vi "LJM_NameToAddress.vi"(8 "error in":errorcluster, 11 "Name":string) -> (0 "error out":errorcluster, 2 "Type":i32, 3 "Address":i32)   [LabVIEW 2025]
uses:
  labjackm.dll
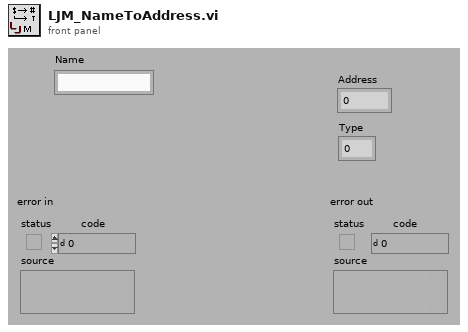
[diagram p1: front panel]
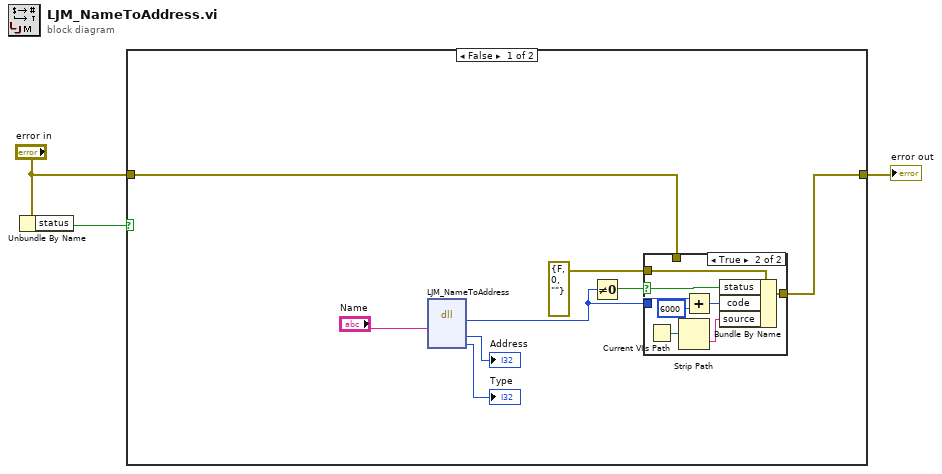
[diagram p0: block diagram]
diagram:
  n1 = Unbundle By Name("error in") -> ("status"=w3:bool)
  n2 = case shown="False" w3 {
    tunnel: "error in" -> [w8 w21]
    tunnel: [w7 w21] -> w1
    frame False {
      n3 = dll-call lib="labjackm.dll" fn="LJM_NameToAddress"("Name"="Name") -> (w11:i32, "Address"=→"Address":i32, "Type"=→"Type":i32)  [unwired: 6 in, 2 out]
      n4 = Not Equal To 0?(x=w11) -> (x != 0?=w10:bool)
      n5 = case shown="True" w10 {
        selector: w10 -> [_ w19]
        tunnel: [w12 w20] -> w7
        tunnel: errorcluster {"status"=FALSE, "code"=0, "source"=""} ("error IO") -> [_ w18]
        tunnel: w11 -> [_ w14]
        tunnel: w8 -> [w12 _]
        frame False {
        }
        frame True {
          n6 = Current VI's Path() -> (path=w16:path)
          n7 = Strip Path(path=w16) -> (name=w17:string)  [unwired: 1 out]
          n8 = Add(x=w14, y=6000) -> (x+y=w15:i32)
          n9 = Bundle By Name(cluster=w18, "status"=w19, "code"=w15, "source"=w17) -> (w20:errorcluster)
        }
      }
    }
    frame True {
    }
  }
  "error out" <- w1
